vi "Process.vi"(8 "error in (no error)":errorcluster, 11 "ADAS PE Template in":refnum<class "ADAS PE Template.lvclass">) -> (0 "error out":errorcluster, 3 "ADAS PE Template out":refnum<class "ADAS PE Template.lvclass">)   [LabVIEW 2020, in "ADAS PE Template.lvlib" / "ADAS PE Template.lvclass"]
doc: "<b>Process</b>\nThis method is called based on the timing set in the <b>Initialize</b> or <b>Configure Session</b> methods, and is where the vast majority of the work done by your plugin will happen. Here, your plugin can read the data that was sent to the plugin (if any), perform some action(s), and optionally send data to the PEF Engine for other plugins to receive.\n\nThe Process state gets called repeatedly by the engine. You do not need to implement a while loop to continuously run in the Process state. Your process state must not call any code with an infinite timeout. \nInstead, use a defined timeout and handle/ignore the timeout error accordingly. This ensures that the system does not hang or get stuck.\n\nThere may be many instances of the same plugin running on the system. Because the state VIs in plugins run with Shared Clone reentrancy, there is no guarantee that any data stored in diagram or front panel structures (such as feedback nodes, shift registers, front panel objects, etc) are from the same instance of the plugin. Any data that needs to persist between calls to the Process VI must be persisted in the class private data of the plugin."
uses:
  ADAS PE Template.lvclass
  C:/Program Files/National Instruments/LabVIEW 2020/vi.lib/FlexLogger/SDK/PluginSDK.lvlibp/PEFClasses/SDK/Processing Element/Processing Element.lvclass
  <vilib>/FlexLogger/SDK/PluginSDK.lvlibp/PEFClasses/SDK/Processing Element/Read System Interface.vi
  <vilib>/FlexLogger/SDK/PluginSDK.lvlibp/PEFClasses/SDK/System Interface/System Interface.lvclass
  ADAS PE Template.lvclass/ADAS PE Template.ctl
  <vilib>/ADAS Record/Utilities/ADAS Utilities.lvlib
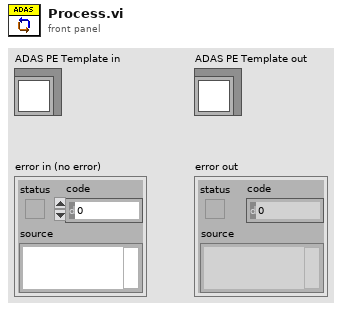
[diagram p1: front panel]
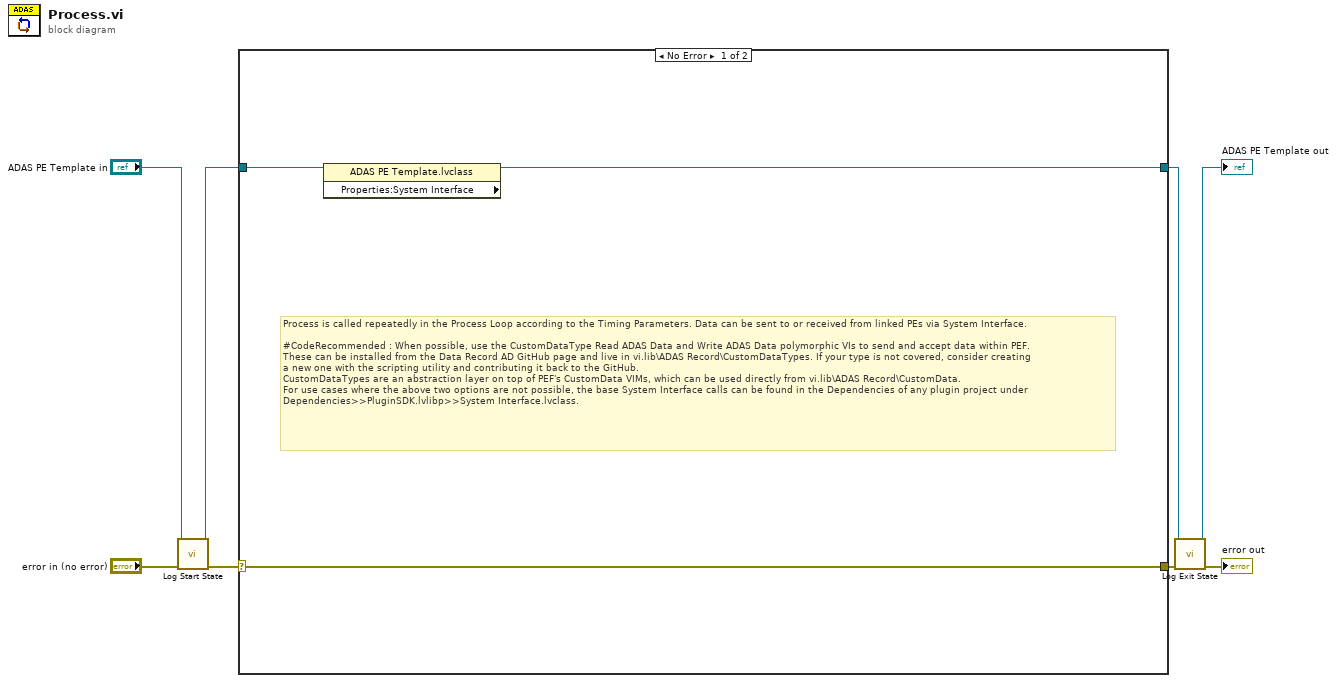
[diagram p0: block diagram]
diagram:
  n1 = call <vilib>:"Log Start State.vi"("error in (no error)"="error in (no error)", "PluginSDK.lvlibp:Processing Element.lvclass"="ADAS PE Template in") -> ("error out"=w7:errorcluster, "PluginSDK.lvlibp:Processing Element.lvclass"=w5:refnum<class "ADAS PE Template.lvclass">)  [unwired: 8 in]
  n2 = case shown="No Error" w7 {
    selector: w7 -> [w9 w12]
    tunnel: [w10 w13] -> w2
    tunnel: w5 -> [w11 w13]
    tunnel: [w9 w12] -> w4
    frame No Error {
      # "Process is called repeatedly in the Process Loop according to the Timing Parameters. Data can be sent to or received from linked PEs via System Interface.\n\n#CodeRecommended : When possible, use the CustomDataType Read ADAS Data and Write ADAS Data polymorphic VIs to send and accept data within PEF.\nThese can be installed from the Data Record AD GitHub page and live in vi.lib\\ADAS Record\\CustomDataTypes. If your type is not covered, consider creating\na new one with the scripting utility and contributing it back to the GitHub.\nCustomDataTypes are an abstraction layer on top of PEF's CustomData VIMs, which can be used directly from vi.lib\\ADAS Record\\CustomData.\nFor use cases where the above two options are not possible, the base System Interface calls can be found in the Dependencies of any plugin project under\nDependencies>>PluginSDK.lvlibp>>System Interface.lvclass."
      n3 = property on="Property Node" class="ADAS PE Template.lvclass" props=["Properties:System Interface"](reference=w11) -> (reference out=w10:refnum<class "ADAS PE Template.lvclass">)  [unwired: 1 in, 2 out]
    }
    frame Error {
    }
  }
  n4 = call <vilib>:"Log Exit State.vi"("error in (no error)"=w4, "PluginSDK.lvlibp:Processing Element.lvclass"=w2) -> ("error out"=→"error out":errorcluster, "PluginSDK.lvlibp:Processing Element.lvclass"=→"ADAS PE Template out":refnum<class "ADAS PE Template.lvclass">)  [unwired: 8 in]
